vi "REPORT_GEAR_save_csv.vi"(8 "error_in":errorcluster) -> (0 "error_out":errorcluster)   [LabVIEW 2019]
uses:
  FGV/REPORTS_records_display/FGV_REPORTS_records_display.ctl
  typedef/REPORT_GEAR_all_info.ctl
  typedef/REPORT_GEAR_header_data_display.ctl
  typedef/REPORT_GEAR_statuses.ctl
  _misc/AULocalize/SubVIs/Get Localized Phrase Compact Interface 0D.vi
  <vilib>/Utility/file.llb/Write Delimited Spreadsheet (string).vi
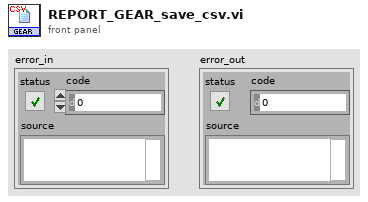
[diagram p1: front panel]
types:
  T1 = typedef "REPORT_GEAR_all_info.ctl" = cluster{"serial":string, "filter_OP":string, "REPORT_GEAR_header":T2, "operations":string[][], "operation_statuses":T3[], "results":string[][], "result_statuses":T3[], "batches":string[][], "batch_statuses":T3[], "column_headers":string[], "displayed_rows":string[][], "displayed_statuses":T3[], "column_widths":i16[]}
  T2 = typedef "REPORT_GEAR_header_data_display.ctl" = cluster{"ID":string, "creation_time":string, "last_station":string, "last_status":string, "pinion_serial":string, "batch_code":string}
  T3 = typedef "REPORT_GEAR_statuses.ctl" = enum16{"OP_OK_hide", "OP_OK_show", "OP_NOK_hide", "OP_NOK_show", "OP_interrupted_hide", "OP_interrupted_show", "OP_in_operation_hide", "OP_in_operation_show", "OP_unexpected_hide", "OP_unexpected_show", "RE_REAL_OK", "RE_REAL_NOK", "RE_STRING", "RE_sub_header", "RE_no_data", "RE_unexpected", "BA_sub_header", "BA_data", "BA_no_data"}
  T4 = typedef "FGV_REPORTS_records_display.ctl" = enum16{"initialize", "GEAR_set_serial", "GEAR_set_header", "GEAR_set_operations", "GEAR_set_results", "GEAR_set_batches", "GEAR_get_serial", "GEAR_get_operation_IDs", "GEAR_toggle_results", "GEAR_show_all_results", "GEAR_hide_all_results", "GEAR_display", "GEAR_filter", "GEAR_restore", "GEAR_clear", "GEAR_get_all_info", "DATES_set_dates", "DATES_set_gears", "DATES_display", "DATES_filter", "DATES_first_page", "DATES_previous_page", "DATES_next_page", "DATES_last_page", "DATES_restore", "DATES_clear", "DATES_get_all_info", "PBATCH_set_batch_no", "PBATCH_set_gears", "PBATCH_display", "PBATCH_filter", "PBATCH_first_page", "PBATCH_previous_page", "PBATCH_next_page", "PBATCH_last_page", "PBATCH_restore", "PBATCH_clear", "PBATCH_get_all_info", "OPRTN_set_OP", "OPRTN_set_dates", "OPRTN_set_gears", "OPRTN_set_hidden_columns", "OPRTN_display", "OPRTN_filter", "OPRTN_filter_no_page_reset", "OPRTN_first_page", "OPRTN_previous_page", "OPRTN_next_page", "OPRTN_last_page", "OPRTN_restore", "OPRTN_clear", "OPRTN_get_all_info", "CFG_set_type", "CFG_set_dates", "CFG_set_records", "CFG_display", "CFG_filter", "CFG_first_page", "CFG_previous_page", "CFG_next_page", "CFG_last_page", "CFG_restore", "CFG_clear", "CFG_get_all_info", "AUDIT_set_dates", "AUDIT_set_records", "AUDIT_display", "AUDIT_filter", "AUDIT_first_page", "AUDIT_previous_page", "AUDIT_next_page", "AUDIT_last_page", "AUDIT_restore", "AUDIT_clear", "AUDIT_get_all_info", "OKNOK_set_dates", "OKNOK_set_records", "OKNOK_display", "OKNOK_restore", "OKNOK_clear", "OKNOK_get_all_info", "REWORKS_set_dates", "REWORKS_set_from_to", "REWORKS_set_records", "REWORKS_display", "REWORKS_filter", "REWORKS_first_page", "REWORKS_previous_page", "REWORKS_next_page", "REWORKS_last_page", "REWORKS_restore", "REWORKS_clear", "REWORKS_get_all_info", "PACE_set_dates", "PACE_set_limits", "PACE_set_records", "PACE_display", "PACE_restore", "PACE_clear", "PACE_get_all_info", "CBATCH_set_code", "CBATCH_set_records", "CBATCH_display", "CBATCH_filter", "CBATCH_first_page", "CBATCH_previous_page", "CBATCH_next_page", "CBATCH_last_page", "CBATCH_restore", "CBATCH_clear", "CBATCH_get_all_info", "CMPNT_set_serial", "CMPNT_set_records", "CMPNT_display", "CMPNT_first_page", "CMPNT_previous_page", "CMPNT_next_page", "CMPNT_last_page", "CMPNT_restore", "CMPNT_clear", "CMPNT_get_all_info", "clear"}
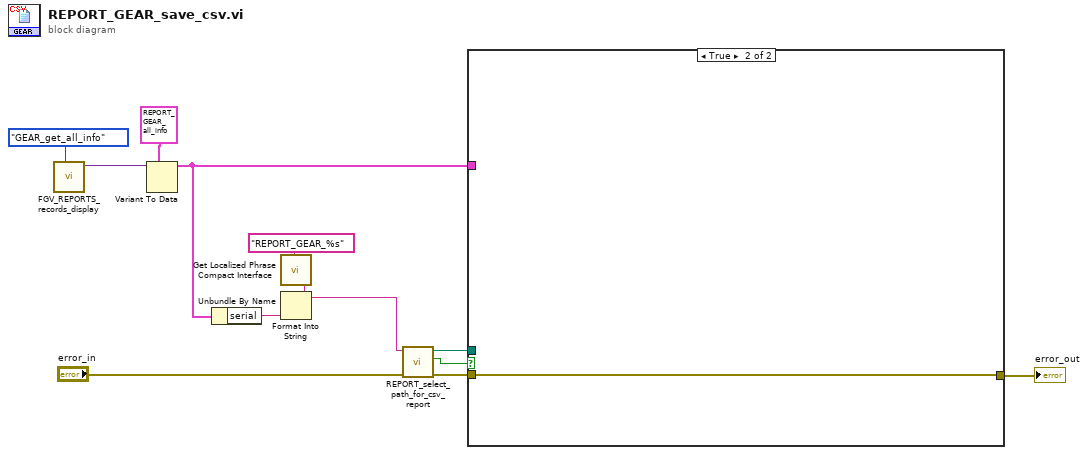
[diagram p0: block diagram]
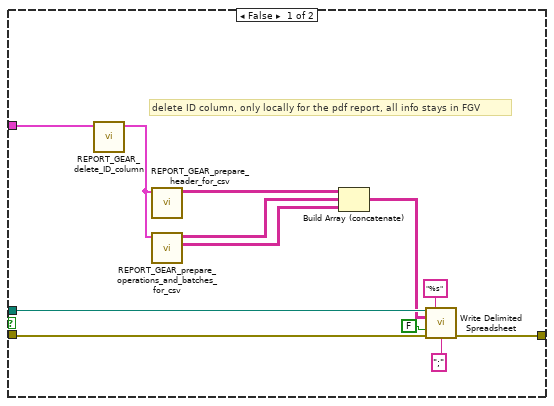
[diagram p2: hidden frame]
diagram:
  n1 = call "FGV_REPORTS_records_display.vi"("options"=FGV_REPORTS_records_display."GEAR_get_all_info") -> ("output"=w12:variant)  [unwired: 9 in, 1 out]
  n2 = Variant To Data(type=T1 {"serial"="", "filter_OP"="", "REPORT_GEAR_header"={"ID"="", "creation_time"="", "last_station"="", "last_status"="", "pinion_serial"="", "batch_code"=""}, "operations"=[], "operation_statuses"=[], "results"=[], "result_statuses"=[], "batches"=[], "batch_statuses"=[], "column_headers"=[], "displayed_rows"=[], "displayed_statuses"=[], "column_widths"=[]} ("REPORT_GEAR_all_info"), Variant=w12) -> (data=w6:T1)  [unwired: 1 in, 1 out]
  n3 = Unbundle By Name(w6) -> ("serial"=w8:string)
  n4 = call-poly "Get Localized Phrase Compact Interface.vi"("Key"="REPORT_GEAR_%s" ("report_title")) -> ("Translated Phrase"=w1:string)
  n5 = Format Into String(format string=w1, w8) -> (resulting string=w7:string)  [unwired: 2 in, 1 out]
  n6 = call "REPORT_select_path_for_csv_report.vi"("error_in"="error_in", "report_title"=w7) -> ("error_out"=w3:errorcluster, "Cancelled?"=w4:bool, "path_to_report"=w5:path)  [unwired: 7 in]
  n7 = case shown="True" w4 {
    tunnel: w6 -> [w25 _]
    tunnel: w5 -> [w23 _]
    tunnel: w3 -> [w15 w26]
    tunnel: [w14 w26] -> w2
    frame False {
      # "delete ID column, only locally for the pdf report, all info stays in FGV"
      n8 = call "REPORT_GEAR_delete_ID_column.vi"("REPORT_GEAR_all_info"=w25) -> ("REPORT_GEAR_all_info_ID_deleted"=w18:T1)  [unwired: 10 in]
      n9 = call "REPORT_GEAR_prepare_header_for_csv.vi"("REPORT_GEAR_all_info"=w18) -> ("report_header"=w20:string[][])  [unwired: 10 in]
      n10 = call "REPORT_GEAR_prepare_operations_and_batches_for_csv.vi"("REPORT_GEAR_all_info"=w18) -> ("report_batches"=w16:string[][], "report_results"=w17:string[][])  [unwired: 9 in]
      n11 = Build Array (concatenate)(w20, w17, w16) -> (w19:string[][])
      n12 = call-poly <vilib>:"Write Delimited Spreadsheet.vi"("file path (dialog if empty)"=w23, "format (%s)"="%s" ("format (%.3f)"), "2D data"=w19, "append to file? (new file:F)"=FALSE, "error in (no error)"=w15, "delimiter (\\t)"=";" ("delimiter (\\t)")) -> ("error out"=w14:errorcluster)  [unwired: 8 in, 1 out]
    }
    frame True {
    }
  }
  "error_out" <- w2
